vi "Get TDMS Reference.vi"(8 "Error In":errorcluster, 11 "LHW-TDMS-Storage-Actor in":refnum<class "LHW-TDMS-Storage-Actor.lvclass">) -> (0 "Error Out":errorcluster, 2 "TDMS Ref":refnum<k34>, 3 "LHW-TDMS-Storage-Actor out":refnum<class "LHW-TDMS-Storage-Actor.lvclass">)   [LabVIEW 2016, in "LHW-TDMS-Storage.lvlib" / "LHW-TDMS-Storage-Actor.lvclass"]
doc: "Return TDMS file reference. Open new file if reference i not valid."
uses:
  LHW-TDMS-Storage-Actor.lvclass
  LHW-TDMS-Storage-Actor.lvclass/LHW-TDMS-Storage-Actor.ctl
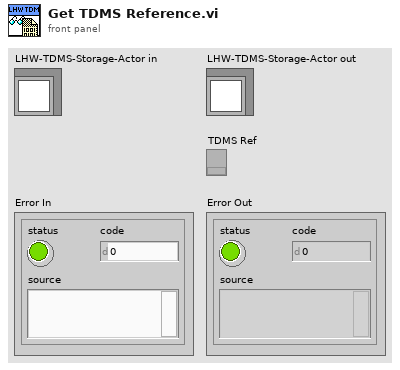
[diagram p1: front panel]
types:
  T1 = enum16{"open", "open or create", "create or replace", "create", "open (read-only)"}
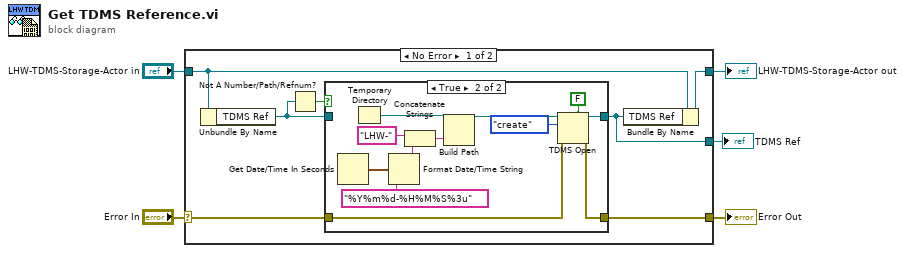
[diagram p0: block diagram]
diagram:
  n1 = case shown="No Error" "Error In" {
    selector: "Error In" -> [w8 w28]
    tunnel: [w7 w28] -> w4
    tunnel: [w9 w27] -> w2
    tunnel: "LHW-TDMS-Storage-Actor in" -> [w10 w27]
    tunnel: [w6 _] -> w1
    frame No Error {
      n2 = Unbundle By Name(w10) -> ("TDMS Ref"=w11:refnum<k34>)
      n3 = Not A Number/Path/Refnum?(number/path/refnum=w11) -> (NaN/Path/Refnum?=w12:bool)
      n4 = case shown="True" w12 {
        tunnel: w11 -> [w14 _]
        tunnel: [w14 w26] -> w6
        tunnel: w8 -> [w13 w25]
        tunnel: [w13 w24] -> w7
        frame False {
        }
        frame True {
          n5 = Get Date/Time In Seconds() -> (seconds since 1Jan1904=w23:timestamp)
          n6 = Temporary Directory() -> (w19:path)
          n7 = Format Date/Time String(time format string (%c)="%Y%m%d-%H%M%S%3u", seconds (now)=w23) -> (date/time string=w20:string)  [unwired: 1 in]
          n8 = Concatenate Strings("LHW-" ("string"), w20) -> (w18:string)
          n9 = Build Path(base path=w19, name or relative path=w18) -> (appended path=w17:path)
          n10 = TDMS Open(5:FALSE ("create index file? (T)"), 8:w25, 10:T1."create" ("operation (0:open)"), 11:w17) -> (0:w24:errorcluster, 3:w26:refnum<k34>)  [unwired: 3 in]
        }
      }
      n11 = Bundle By Name(cluster=w10, "TDMS Ref"=w6) -> (w9:refnum<class "LHW-TDMS-Storage-Actor.lvclass">)
    }
    frame Error {
    }
  }
  "Error Out" <- w4
  "LHW-TDMS-Storage-Actor out" <- w2
  "TDMS Ref" <- w1
